vi "nanocal -- nuclear schottky fit V5.vi"() -> ()   [LabVIEW 2020] (continued)
"IDS0323_210901_RAW_cal__ref_"="IDS0323_210901_RAW_cal_CeCoIn5_4th_052(138)_C(f)_12T_3.10K_45deg_Tdep_raw_.dat", "IDS0323_210901_RAW_cal__sam_"="IDS0323_210901_RAW_cal_CeCoIn5_4th_052(138)_C(f)_12T_3.10K_45deg_Tdep_raw_.dat", "IDS0324_210901_RAW_cal__ref_"="IDS0324_210901_RAW_cal_CeCoIn5_4th_053(139)_C(f)_12T_5.70K_45deg_Tdep_raw_.dat", "IDS0324_210901_RAW_cal__sam_"="IDS0324_210901_RAW_cal_CeCoIn5_4th_053(139)_C(f)_12T_5.70K_45deg_Tdep_raw_.dat", "IDS0330_210901_RAW_cal__ref_"="IDS0330_210901_RAW_cal_CeCoIn5_4th_059_C(f)_1T_0.197K_90deg_Bdep_raw_.dat", "IDS0330_210901_RAW_cal__sam_"="IDS0330_210901_RAW_cal_CeCoIn5_4th_059_C(f)_1T_0.197K_90deg_Bdep_raw_.dat", "IDS0331_210901_RAW_cal__ref_"="IDS0331_210901_RAW_cal_CeCoIn5_4th_060_C(f)_2T_0.197K_90deg_Bdep_raw_.dat", "IDS0331_210901_RAW_cal__sam_"="IDS0331_210901_RAW_cal_CeCoIn5_4th_060_C(f)_2T_0.197K_90deg_Bdep_raw_.dat", "IDS0335_210904_RAW_cal__ref_"="IDS0335_210904_RAW_cal_CeCoIn5_4th_064_C(f)_5.0T_0.197K_90deg_fsweep_Tdep_raw_.dat", "IDS0335_210904_RAW_cal__sam_"="IDS0335_210904_RAW_cal_CeCoIn5_4th_064_C(f)_5.0T_0.197K_90deg_fsweep_Tdep_raw_.dat", "IDS0336_210904_RAW_cal__ref_"="IDS0336_210904_RAW_cal_CeCoIn5_4th_065_C(f)_5.0T_0.122K_90deg_fsweep_Tdep_raw_.dat", "IDS0336_210904_RAW_cal__sam_"="IDS0336_210904_RAW_cal_CeCoIn5_4th_065_C(f)_5.0T_0.122K_90deg_fsweep_Tdep_raw_.dat", "IDS0337_210904_RAW_cal__ref_"="IDS0337_210904_RAW_cal_CeCoIn5_4th_066_C(f)_5.0T_0.157K_90deg_Tdep_raw_.dat", "IDS0337_210904_RAW_cal__sam_"="IDS0337_210904_RAW_cal_CeCoIn5_4th_066_C(f)_5.0T_0.157K_90deg_Tdep_raw_.dat", "IDS0338_210904_RAW_cal__ref_"="IDS0338_210904_RAW_cal_CeCoIn5_4th_067_C(f)_5.0T_0.170K_90deg_Tdep_raw_.dat", "IDS0338_210904_RAW_cal__sam_"="IDS0338_210904_RAW_cal_CeCoIn5_4th_067_C(f)_5.0T_0.170K_90deg_Tdep_raw_.dat", "IDS0339_210904_RAW_cal__ref_"="IDS0339_210904_RAW_cal_CeCoIn5_4th_068_C(f)_5.0T_0.255K_90deg_Tdep_raw_.dat", "IDS0339_210904_RAW_cal__sam_"="IDS0339_210904_RAW_cal_CeCoIn5_4th_068_C(f)_5.0T_0.255K_90deg_Tdep_raw_.dat", "IDS0340_210904_RAW_cal__ref_"="IDS0340_210904_RAW_cal_CeCoIn5_4th_069_C(f)_5.0T_0.308K_90deg_Tdep_raw_.dat", "IDS0340_210904_RAW_cal__sam_"="IDS0340_210904_RAW_cal_CeCoIn5_4th_069_C(f)_5.0T_0.308K_90deg_Tdep_raw_.dat", "IDS0341_210904_RAW_cal__ref_"="IDS0341_210904_RAW_cal_CeCoIn5_4th_070_C(f)_5.0T_0.360K_90deg_Tdep_raw_.dat", "IDS0341_210904_RAW_cal__sam_"="IDS0341_210904_RAW_cal_CeCoIn5_4th_070_C(f)_5.0T_0.360K_90deg_Tdep_raw_.dat", "IDS0342_210904_RAW_cal__ref_"="IDS0342_210904_RAW_cal_CeCoIn5_4th_071_C(f)_5.0T_0.438K_90deg_Tdep_raw_.dat", "IDS0342_210904_RAW_cal__sam_"="IDS0342_210904_RAW_cal_CeCoIn5_4th_071_C(f)_5.0T_0.438K_90deg_Tdep_raw_.dat", "IDS0343_210904_RAW_cal__ref_"="IDS0343_210904_RAW_cal_CeCoIn5_4th_072_C(f)_5.0T_0.53K_90deg_Tdep_raw_.dat", "IDS0343_210904_RAW_cal__sam_"="IDS0343_210904_RAW_cal_CeCoIn5_4th_072_C(f)_5.0T_0.53K_90deg_Tdep_raw_.dat", "IDS0344_210904_RAW_cal__ref_"="IDS0344_210904_RAW_cal_CeCoIn5_4th_073_C(f)_5.0T_0.62K_90deg_Tdep_raw_.dat", "IDS0344_210904_RAW_cal__sam_"="IDS0344_210904_RAW_cal_CeCoIn5_4th_073_C(f)_5.0T_0.62K_90deg_Tdep_raw_.dat", "IDS0346_210904_RAW_cal__ref_"="IDS0346_210904_RAW_cal_CeCoIn5_4th_075_C(f)_8.0T_0.122K_90deg_Tdep_raw_.dat", "IDS0346_210904_RAW_cal__sam_"="IDS0346_210904_RAW_cal_CeCoIn5_4th_075_C(f)_8.0T_0.122K_90deg_Tdep_raw_.dat", "IDS0347_210906_RAW_cal__ref_"="IDS0347_210906_RAW_cal_CeCoIn5_4th_076_C(f)_8.0T_0.157K_90deg_Tdep_raw_.dat", "IDS0347_210906_RAW_cal__sam_"="IDS0347_210906_RAW_cal_CeCoIn5_4th_076_C(f)_8.0T_0.157K_90deg_Tdep_raw_.dat", "IDS0348_210906_RAW_cal__ref_"="IDS0348_210906_RAW_cal_CeCoIn5_4th_077_C(f)_8.0T_0.178K_90deg_Tdep_raw_.dat", "IDS0348_210906_RAW_cal__sam_"="IDS0348_210906_RAW_cal_CeCoIn5_4th_077_C(f)_8.0T_0.178K_90deg_Tdep_raw_.dat", "IDS0349_210906_RAW_cal__ref_"="IDS0349_210906_RAW_cal_CeCoIn5_4th_078_C(f)_8.0T_0.20K_90deg_Tdep_raw_.dat", "IDS0349_210906_RAW_cal__sam_"="IDS0349_210906_RAW_cal_CeCoIn5_4th_078_C(f)_8.0T_0.20K_90deg_Tdep_raw_.dat", "IDS0350_210906_RAW_cal__ref_"="IDS0350_210906_RAW_cal_CeCoIn5_4th_079_C(f)_8.0T_0.26K_90deg_Tdep_raw_.dat", "IDS0350_210906_RAW_cal__sam_"="IDS0350_210906_RAW_cal_CeCoIn5_4th_079_C(f)_8.0T_0.26K_90deg_Tdep_raw_.dat", "IDS0351_210906_RAW_cal__ref_"="IDS0351_210906_RAW_cal_CeCoIn5_4th_080_C(f)_8.0T_0.31K_90deg_Tdep_raw_.dat", "IDS0351_210906_RAW_cal__sam_"="IDS0351_210906_RAW_cal_CeCoIn5_4th_080_C(f)_8.0T_0.31K_90deg_Tdep_raw_.dat", "IDS0352_210906_RAW_cal__ref_"="IDS0352_210906_RAW_cal_CeCoIn5_4th_081_C(f)_8.0T_0.36K_90deg_Tdep_raw_.dat", "IDS0352_210906_RAW_cal__sam_"="IDS0352_210906_RAW_cal_CeCoIn5_4th_081_C(f)_8.0T_0.36K_90deg_Tdep_raw_.dat", "IDS0353_210906_RAW_cal__ref_"="IDS0353_210906_RAW_cal_CeCoIn5_4th_082_C(f)_8.0T_0.438K_90deg_Tdep_raw_.dat", "IDS0353_210906_RAW_cal__sam_"="IDS0353_210906_RAW_cal_CeCoIn5_4th_082_C(f)_8.0T_0.438K_90deg_Tdep_raw_.dat", "IDS0354_210906_RAW_cal__ref_"="IDS0354_210906_RAW_cal_CeCoIn5_4th_083_C(f)_8.0T_0.53K_90deg_Tdep_raw_.dat", "IDS0354_210906_RAW_cal__sam_"="IDS0354_210906_RAW_cal_CeCoIn5_4th_083_C(f)_8.0T_0.53K_90deg_Tdep_raw_.dat", "IDS0355_210906_RAW_cal__ref_"="IDS0355_210906_RAW_cal_CeCoIn5_4th_085_C(f)_8.0T_0.83K_90deg_Tdep_raw_.dat", "IDS0355_210906_RAW_cal__sam_"="IDS0355_210906_RAW_cal_CeCoIn5_4th_085_C(f)_8.0T_0.83K_90deg_Tdep_raw_.dat", "IDS0359_210907_RAW_cal__ref_"="IDS0359_210907_RAW_cal_CeCoIn5_4th_089_C(f)_12.0T_0.12K_60deg_Tdep_raw_.dat", "IDS0359_210907_RAW_cal__sam_"="IDS0359_210907_RAW_cal_CeCoIn5_4th_089_C(f)_12.0T_0.12K_60deg_Tdep_raw_.dat", "IDS0360_210907_RAW_cal__ref_"="IDS0360_210907_RAW_cal_CeCoIn5_4th_090_C(f)_12.0T_0.15K_60deg_Tdep_raw_.dat", "IDS0360_210907_RAW_cal__sam_"="IDS0360_210907_RAW_cal_CeCoIn5_4th_090_C(f)_12.0T_0.15K_60deg_Tdep_raw_.dat", "IDS0361_210908_RAW_cal__ref_"="IDS0361_210908_RAW_cal_CeCoIn5_4th_091_C(f)_12.0T_0.168K_60deg_Tdep_raw_.dat", "IDS0361_210908_RAW_cal__sam_"="IDS0361_210908_RAW_cal_CeCoIn5_4th_091_C(f)_12.0T_0.168K_60deg_Tdep_raw_.dat", "IDS0362_210908_RAW_cal__ref_"="IDS0362_210908_RAW_cal_CeCoIn5_4th_092_C(f)_12.0T_0.197K_60deg_Tdep_raw_.dat", "IDS0362_210908_RAW_cal__sam_"="IDS0362_210908_RAW_cal_CeCoIn5_4th_092_C(f)_12.0T_0.197K_60deg_Tdep_raw_.dat", "IDS0363_210908_RAW_cal__ref_"="IDS0363_210908_RAW_cal_CeCoIn5_4th_093_C(f)_12.0T_0.25K_60deg_Tdep_raw_.dat", "IDS0363_210908_RAW_cal__sam_"="IDS0363_210908_RAW_cal_CeCoIn5_4th_093_C(f)_12.0T_0.25K_60deg_Tdep_raw_.dat", "IDS0364_210908_RAW_cal__ref_"="IDS0364_210908_RAW_cal_CeCoIn5_4th_094_C(f)_12.0T_0.307K_60deg_Tdep_raw_.dat", "IDS0364_210908_RAW_cal__sam_"="IDS0364_210908_RAW_cal_CeCoIn5_4th_094_C(f)_12.0T_0.307K_60deg_Tdep_raw_.dat", "IDS0365_210908_RAW_cal__ref_"="IDS0365_210908_RAW_cal_CeCoIn5_4th_095_C(f)_12.0T_0.36K_60deg_Tdep_raw_.dat", "IDS0365_210908_RAW_cal__sam_"="IDS0365_210908_RAW_cal_CeCoIn5_4th_095_C(f)_12.0T_0.36K_60deg_Tdep_raw_.dat", "IDS0366_210908_RAW_cal__ref_"="IDS0366_210908_RAW_cal_CeCoIn5_4th_096_C(f)_12.0T_0.43K_60deg_Tdep_raw_.dat", "IDS0366_210908_RAW_cal__sam_"="IDS0366_210908_RAW_cal_CeCoIn5_4th_096_C(f)_12.0T_0.43K_60deg_Tdep_raw_.dat", "IDS0367_210908_RAW_cal__ref_"="IDS0367_210908_RAW_cal_CeCoIn5_4th_097_C(f)_12.0T_0.53K_60deg_Tdep_raw_.dat", "IDS0367_210908_RAW_cal__sam_"="IDS0367_210908_RAW_cal_CeCoIn5_4th_097_C(f)_12.0T_0.53K_60deg_Tdep_raw_.dat", "IDS0368_210908_RAW_cal__ref_"="IDS0368_210908_RAW_cal_CeCoIn5_4th_098_C(f)_12.0T_0.63K_60deg_Tdep_raw_.dat", "IDS0368_210908_RAW_cal__sam_"="IDS0368_210908_RAW_cal_CeCoIn5_4th_098_C(f)_12.0T_0.63K_60deg_Tdep_raw_.dat", "IDS0369_210908_RAW_cal__ref_"="IDS0369_210908_RAW_cal_CeCoIn5_4th_099_C(f)_12.0T_0.83K_60deg_Tdep_raw_.dat", "IDS0369_210908_RAW_cal__sam_"="IDS0369_210908_RAW_cal_CeCoIn5_4th_099_C(f)_12.0T_0.83K_60deg_Tdep_raw_.dat", "IDS0370_210908_RAW_cal__ref_"="IDS0370_210908_RAW_cal_CeCoIn5_4th_100_C(f)_12.0T_1.13K_60deg_Tdep_raw_.dat", "IDS0370_210908_RAW_cal__sam_"="IDS0370_210908_RAW_cal_CeCoIn5_4th_100_C(f)_12.0T_1.13K_60deg_Tdep_raw_.dat", "IDS0371_210908_RAW_cal__ref_"="IDS0371_210908_RAW_cal_CeCoIn5_4th_101_C(f)_12.0T_1.90K_60deg_Tdep_raw_.dat", "IDS0371_210908_RAW_cal__sam_"="IDS0371_210908_RAW_cal_CeCoIn5_4th_101_C(f)_12.0T_1.90K_60deg_Tdep_raw_.dat", "IDS0372_210908_RAW_cal__ref_"="IDS0372_210908_RAW_cal_CeCoIn5_4th_102_C(f)_12.0T_3.11K_60deg_Tdep_raw_.dat", "IDS0372_210908_RAW_cal__sam_"="IDS0372_210908_RAW_cal_CeCoIn5_4th_102_C(f)_12.0T_3.11K_60deg_Tdep_raw_.dat", "IDS0373_210908_RAW_cal__ref_"="IDS0373_210908_RAW_cal_CeCoIn5_4th_103_C(f)_12.0T_5.75K_60deg_Tdep_raw_.dat", "IDS0373_210908_RAW_cal__sam_"="IDS0373_210908_RAW_cal_CeCoIn5_4th_103_C(f)_12.0T_5.75K_60deg_Tdep_raw_.dat", "IDS0377_210909_RAW_cal__ref_"="IDS0377_210909_RAW_cal_CeCoIn5_4th_107_C(f)_8.0T_0.197K_0deg_Tdep_raw_.dat", "IDS0377_210909_RAW_cal__sam_"="IDS0377_210909_RAW_cal_CeCoIn5_4th_107_C(f)_8.0T_0.197K_0deg_Tdep_raw_.dat", "IDS0378_210909_RAW_cal__ref_"="IDS0378_210909_RAW_cal_CeCoIn5_4th_108_C(f)_8.0T_0.122K_0deg_Tdep_raw_.dat", "IDS0378_210909_RAW_cal__sam_"="IDS0378_210909_RAW_cal_CeCoIn5_4th_108_C(f)_8.0T_0.122K_0deg_Tdep_raw_.dat", "IDS0379_210909_RAW_cal__ref_"="IDS0379_210909_RAW_cal_CeCoIn5_4th_109_C(f)_8.0T_0.148K_0deg_Tdep_raw_.dat", "IDS0379_210909_RAW_cal__sam_"="IDS0379_210909_RAW_cal_CeCoIn5_4th_109_C(f)_8.0T_0.148K_0deg_Tdep_raw_.dat", "IDS0380_210909_RAW_cal__ref_"="IDS0380_210909_RAW_cal_CeCoIn5_4th_110_C(f)_8.0T_0.168K_0deg_Tdep_raw_.dat", "IDS0380_210909_RAW_cal__sam_"="IDS0380_210909_RAW_cal_CeCoIn5_4th_110_C(f)_8.0T_0.168K_0deg_Tdep_raw_.dat", "IDS0381_210909_RAW_cal__ref_"="IDS0381_210909_RAW_cal_CeCoIn5_4th_111_C(f)_8.0T_0.25K_0deg_Tdep_raw_.dat", "IDS0381_210909_RAW_cal__sam_"="IDS0381_210909_RAW_cal_CeCoIn5_4th_111_C(f)_8.0T_0.25K_0deg_Tdep_raw_.dat", "IDS0382_210909_RAW_cal__ref_"="IDS0382_210909_RAW_cal_CeCoIn5_4th_112_C(f)_8.0T_0.30K_0deg_Tdep_raw_.dat", "IDS0382_210909_RAW_cal__sam_"="IDS0382_210909_RAW_cal_CeCoIn5_4th_112_C(f)_8.0T_0.30K_0deg_Tdep_raw_.dat", "IDS0383_210910_RAW_cal__ref_"="IDS0383_210910_RAW_cal_CeCoIn5_4th_113_C(f)_8.0T_0.36K_0deg_Tdep_raw_.dat", "IDS0383_210910_RAW_cal__sam_"="IDS0383_210910_RAW_cal_CeCoIn5_4th_113_C(f)_8.0T_0.36K_0deg_Tdep_raw_.dat", "IDS0384_210910_RAW_cal__ref_"="IDS0384_210910_RAW_cal_CeCoIn5_4th_114_C(f)_8.0T_0.43K_0deg_Tdep_raw_.dat", "IDS0384_210910_RAW_cal__sam_"="IDS0384_210910_RAW_cal_CeCoIn5_4th_114_C(f)_8.0T_0.43K_0deg_Tdep_raw_.dat", "IDS0385_210910_RAW_cal__ref_"="IDS0385_210910_RAW_cal_CeCoIn5_4th_115_C(f)_8.0T_0.53K_0deg_Tdep_raw_.dat", "IDS0385_210910_RAW_cal__sam_"="IDS0385_210910_RAW_cal_CeCoIn5_4th_115_C(f)_8.0T_0.53K_0deg_Tdep_raw_.dat", "IDS0386_210910_RAW_cal__ref_"="IDS0386_210910_RAW_cal_CeCoIn5_4th_116_C(f)_8.0T_0.63K_0deg_Tdep_raw_.dat", "IDS0386_210910_RAW_cal__sam_"="IDS0386_210910_RAW_cal_CeCoIn5_4th_116_C(f)_8.0T_0.63K_0deg_Tdep_raw_.dat", "IDS0387_210910_RAW_cal__ref_"="IDS0387_210910_RAW_cal_CeCoIn5_4th_117_C(f)_8.0T_0.83K_0deg_Tdep_raw_.dat", "IDS0387_210910_RAW_cal__sam_"="IDS0387_210910_RAW_cal_CeCoIn5_4th_117_C(f)_8.0T_0.83K_0deg_Tdep_raw_.dat", "IDS0388_210910_RAW_cal__ref_"="IDS0388_210910_RAW_cal_CeCoIn5_4th_118_C(f)_8.0T_1.13K_0deg_Tdep_raw_.dat", "IDS0388_210910_RAW_cal__sam_"="IDS0388_210910_RAW_cal_CeCoIn5_4th_118_C(f)_8.0T_1.13K_0deg_Tdep_raw_.dat", "IDS0389_210910_RAW_cal__ref_"="IDS0389_210910_RAW_cal_CeCoIn5_4th_119_C(f)_8.0T_1.52K_0deg_Tdep_raw_.dat", "IDS0389_210910_RAW_cal__sam_"="IDS0389_210910_RAW_cal_CeCoIn5_4th_119_C(f)_8.0T_1.52K_0deg_Tdep_raw_.dat", "IDS0390_210910_RAW_cal__ref_"="IDS0390_210910_RAW_cal_CeCoIn5_4th_120_C(f)_8.0T_1.90K_0deg_Tdep_raw_.dat", "IDS0390_210910_RAW_cal__sam_"="IDS0390_210910_RAW_cal_CeCoIn5_4th_120_C(f)_8.0T_1.90K_0deg_Tdep_raw_.dat", "IDS0391_210910_RAW_cal__ref_"="IDS0391_210910_RAW_cal_CeCoIn5_4th_121_C(f)_8.0T_1.25K_0deg_Tdep_raw_.dat", "IDS0391_210910_RAW_cal__sam_"="IDS0391_210910_RAW_cal_CeCoIn5_4th_121_C(f)_8.0T_1.25K_0deg_Tdep_raw_.dat", "IDS0392_210910_RAW_cal__ref_"="IDS0392_210910_RAW_cal_CeCoIn5_4th_122_C(f)_8.0T_1.39K_0deg_Tdep_raw_.dat", "IDS0392_210910_RAW_cal__sam_"="IDS0392_210910_RAW_cal_CeCoIn5_4th_122_C(f)_8.0T_1.39K_0deg_Tdep_raw_.dat", "IDS0393_210910_RAW_cal__ref_"="IDS0393_210910_RAW_cal_CeCoIn5_4th_123_C(f)_8.0T_3.11K_0deg_Tdep_raw_.dat", "IDS0393_210910_RAW_cal__sam_"="IDS0393_210910_RAW_cal_CeCoIn5_4th_123_C(f)_8.0T_3.11K_0deg_Tdep_raw_.dat", "IDS0394_210910_RAW_cal__ref_"="IDS0394_210910_RAW_cal_CeCoIn5_4th_124_C(f)_8.0T_5.75K_0deg_Tdep_raw_.dat", "IDS0394_210910_RAW_cal__sam_"="IDS0394_210910_RAW_cal_CeCoIn5_4th_124_C(f)_8.0T_5.75K_0deg_Tdep_raw_.dat", "IDS0395_210910_RAW_cal__ref_"="IDS0395_210910_RAW_cal_CeCoIn5_4th_125_C(f)_8.0T_1.31K_0deg_Tdep_raw_.dat", "IDS0395_210910_RAW_cal__sam_"="IDS0395_210910_RAW_cal_CeCoIn5_4th_125_C(f)_8.0T_1.31K_0deg_Tdep_raw_.dat"}
  out "temps&degs":map{string, map{T4, dbl}}(c390)
  out "mathematica thing":map{string, map{T4, dbl}}(c390)
  out "constrained filename lookup":map{i32, string}(c390)={0="IDS0336_210904_RAW_cal__ref_", 1="IDS0337_210904_RAW_cal__ref_", 2="IDS0338_210904_RAW_cal__ref_", 3="IDS0335_210904_RAW_cal__ref_", 4="IDS0339_210904_RAW_cal__ref_", 5="IDS0340_210904_RAW_cal__ref_", 6="IDS0341_210904_RAW_cal__ref_", 7="IDS0342_210904_RAW_cal__ref_", 8="IDS0343_210904_RAW_cal__ref_", 9="IDS0344_210904_RAW_cal__ref_"}
  out "filesnames lookup":map{i32, string}(c390)={0="IDS0183_210310_RAW_cal__sam_", 1="IDS0311_210901_RAW_cal__sam_", 2="IDS0359_210907_RAW_cal__sam_", 3="IDS0336_210904_RAW_cal__sam_", 4="IDS0346_210904_RAW_cal__sam_", 5="IDS0378_210909_RAW_cal__sam_", 6="IDS0158_210310_RAW_cal__sam_", 7="IDS0300_210427_RAW_cal__sam_", 8="IDS0184_210310_RAW_cal__sam_", 9="IDS0210_210310_RAW_cal__sam_", 10="IDS0379_210909_RAW_cal__sam_", 11="IDS0360_210907_RAW_cal__sam_", 12="IDS0310_210901_RAW_cal__sam_", 13="IDS0337_210904_RAW_cal__sam_", 14="IDS0347_210906_RAW_cal__sam_", 15="IDS0305_210831_RAW_cal__sam_", 16="IDS0361_210908_RAW_cal__sam_", 17="IDS0380_210909_RAW_cal__sam_", 18="IDS0159_210310_RAW_cal__sam_", 19="IDS0304_210831_RAW_cal__sam_", 20="IDS0312_210901_RAW_cal__sam_", 21="IDS0338_210904_RAW_cal__sam_", 22="IDS0348_210906_RAW_cal__sam_", 23="IDS0181_210310_RAW_cal__sam_", 24="IDS0185_210310_RAW_cal__sam_", 25="IDS0208_210310_RAW_cal__sam_", 26="IDS0209_210310_RAW_cal__sam_", 27="IDS0211_210310_RAW_cal__sam_", 28="IDS0212_210310_RAW_cal__sam_", 29="IDS0213_210310_RAW_cal__sam_", 30="IDS0214_210310_RAW_cal__sam_", 31="IDS0215_210310_RAW_cal__sam_", 32="IDS0216_210310_RAW_cal__sam_", 33="IDS0217_210310_RAW_cal__sam_", 34="IDS0330_210901_RAW_cal__sam_", 35="IDS0331_210901_RAW_cal__sam_", 36="IDS0335_210904_RAW_cal__sam_", 37="IDS0362_210908_RAW_cal__sam_", 38="IDS0377_210909_RAW_cal__sam_", 39="IDS0160_210310_RAW_cal__sam_", 40="IDS0303_210831_RAW_cal__sam_", 41="IDS0313_210901_RAW_cal__sam_", 42="IDS0349_210906_RAW_cal__sam_", 43="IDS0161_210310_RAW_cal__sam_", 44="IDS0186_210310_RAW_cal__sam_", 45="IDS0302_210831_RAW_cal__sam_", 46="IDS0363_210908_RAW_cal__sam_", 47="IDS0381_210909_RAW_cal__sam_", 48="IDS0314_210901_RAW_cal__sam_", 49="IDS0339_210904_RAW_cal__sam_", 50="IDS0350_210906_RAW_cal__sam_", 51="IDS0162_210310_RAW_cal__sam_", 52="IDS0187_210310_RAW_cal__sam_", 53="IDS0301_210831_RAW_cal__sam_", 54="IDS0315_210901_RAW_cal__sam_", 55="IDS0382_210909_RAW_cal__sam_", 56="IDS0364_210908_RAW_cal__sam_", 57="IDS0340_210904_RAW_cal__sam_", 58="IDS0351_210906_RAW_cal__sam_", 59="IDS0163_210310_RAW_cal__sam_", 60="IDS0188_210310_RAW_cal__sam_", 61="IDS0299_210427_RAW_cal__sam_", 62="IDS0316_210901_RAW_cal__sam_", 63="IDS0341_210904_RAW_cal__sam_", 64="IDS0352_210906_RAW_cal__sam_", 65="IDS0365_210908_RAW_cal__sam_", 66="IDS0383_210910_RAW_cal__sam_", 67="IDS0164_210310_RAW_cal__sam_", 68="IDS0189_210310_RAW_cal__sam_", 69="IDS0298_210427_RAW_cal__sam_", 70="IDS0317_210901_RAW_cal__sam_", 71="IDS0366_210908_RAW_cal__sam_", 72="IDS0384_210910_RAW_cal__sam_", 73="IDS0342_210904_RAW_cal__sam_", 74="IDS0353_210906_RAW_cal__sam_", 75="IDS0165_210310_RAW_cal__sam_", 76="IDS0190_210310_RAW_cal__sam_", 77="IDS0297_210427_RAW_cal__sam_", 78="IDS0318_210901_RAW_cal__sam_", 79="IDS0343_210904_RAW_cal__sam_", 80="IDS0354_210906_RAW_cal__sam_", 81="IDS0367_210908_RAW_cal__sam_", 82="IDS0385_210910_RAW_cal__sam_", 83="IDS0166_210310_RAW_cal__sam_", 84="IDS0191_210310_RAW_cal__sam_", 85="IDS0296_210427_RAW_cal__sam_", 86="IDS0319_210901_RAW_cal__sam_", 87="IDS0344_210904_RAW_cal__sam_", 88="IDS0368_210908_RAW_cal__sam_", 89="IDS0386_210910_RAW_cal__sam_", 90="IDS0220_210310_RAW_cal__sam_", 91="IDS0167_210310_RAW_cal__sam_", 92="IDS0192_210310_RAW_cal__sam_", 93="IDS0295_210427_RAW_cal__sam_", 94="IDS0320_210901_RAW_cal__sam_", 95="IDS0355_210906_RAW_cal__sam_", 96="IDS0369_210908_RAW_cal__sam_", 97="IDS0387_210910_RAW_cal__sam_", 98="IDS0168_210310_RAW_cal__sam_", 99="IDS0219_210310_RAW_cal__sam_", 100="IDS0193_210310_RAW_cal__sam_", 101="IDS0294_210427_RAW_cal__sam_", 102="IDS0321_210901_RAW_cal__sam_", 103="IDS0370_210908_RAW_cal__sam_", 104="IDS0388_210910_RAW_cal__sam_", 105="IDS0169_210310_RAW_cal__sam_", 106="IDS0391_210910_RAW_cal__sam_", 107="IDS0395_210910_RAW_cal__sam_", 108="IDS0392_210910_RAW_cal__sam_", 109="IDS0389_210910_RAW_cal__sam_", 110="IDS0218_210310_RAW_cal__sam_", 111="IDS0194_210310_RAW_cal__sam_", 112="IDS0293_210427_RAW_cal__sam_", 113="IDS0322_210901_RAW_cal__sam_", 114="IDS0371_210908_RAW_cal__sam_", 115="IDS0390_210910_RAW_cal__sam_", 116="IDS0170_210310_RAW_cal__sam_", 117="IDS0195_210310_RAW_cal__sam_", 118="IDS0306_210831_RAW_cal__sam_", 119="IDS0323_210901_RAW_cal__sam_", 120="IDS0372_210908_RAW_cal__sam_", 121="IDS0393_210910_RAW_cal__sam_", 122="IDS0171_210310_RAW_cal__sam_", 123="IDS0196_210310_RAW_cal__sam_", 124="IDS0324_210901_RAW_cal__sam_", 125="IDS0373_210908_RAW_cal__sam_", 126="IDS0394_210910_RAW_cal__sam_", 127="IDS0172_210310_RAW_cal__sam_"}
  in  "parameter map":map{T4, dbl}(c390)={enum."ζ"=0.2919164673041952, enum."τ1"=0.04813472468486327, enum."τS"=0.13257313400894957, enum."τN"=0.017459219246992615, enum."τC"=0.0011273379303887484, enum."κ0"=6.401291929673956e-10}
  out "all full filenames":map{string, path}(c390)
  in  "tab 9":enum32{"Page 1"}(tab)
  in  "# plot steps":i32=200
  out "Plot: oscillations":cluster{"Array":i32[], "Array":dbl[]}(graph)={"Array"=[0, 1, 2, 3, 4, 5, 6, 7, 8, 9, 10, 11, 12, 13, 14, 15, 16, 17, 18, 19, 20, 21, 22, 23, 24, 25, 26, 27, 28, 29, 30, 31, 32, 33, 34, 35, 36, 37, 38, 39, 40, 41, 42, 43, 44, 45, 46, 47, 48, 49, 50, 51, 52, 53, 54, 55, 56, 57, 58, 59, 60, 61, 62, 63, 64, 65, 66, 67, 68, 69, 70, 71, 72, 73, 74, 75, 76, 77, 78, 79, 80, 81, 82, 83, 84, 85, 86, 87, 88, 89, 90, 91, 92, 93, 94, 95, 96, 97, 98, 99, 100, 101, 102, 103, 104, 105, 106, 107, 108, 109, 110, 111, 112, 113, 114, 115, 116, 117, 118, 119, 120, 121, 122, 123, 124, 125, 126, 127, 128, 129, 130, 131, 132, 133, 134, 135, 136, 137, 138, 139, 140, 141, 142, 143, 144, 145, 146, 147, 148, 149, 150, 151, 152, 153, 154, 155, 156, 157, 158, 159, 160, 161, 162, 163, 164, 165, 166, 167, 168, 169, 170, 171, 172, 173, 174, 175, 176, 177, 178, 179, 180, 181, 182, 183, 184, 185, 186, 187, 188, 189, 190, 191, 192, 193, 194, 195, 196, 197, 198, 199], "Array"=[4.450467078198628e-11, 4.3160530704966504e-11, 4.183009494340695e-11, 4.0513266352792954e-11, 3.9210031055336714e-11, 3.792043068440165e-11, 3.664459014007804e-11, 3.5382301255548754e-11, 3.413366811422236e-11, 3.2898669899417143e-11, 3.167733436670872e-11, 3.0469723966142226e-11, 2.927564440868835e-11, 2.8095047122089767e-11, 2.6928285989935574e-11, 2.5775048762000097e-11, 2.4635564421782163e-11, 2.3509562352419522e-11, 2.239730623188052e-11, 2.1298608710029754e-11, 2.0213615503639204e-11, 1.9142160079255177e-11, 1.8084339581392328e-11, 1.704010543779333e-11, 1.600961724301797e-11, 1.4992611319097904e-11, 1.3989330527319765e-11, 1.2999573639760342e-11, 1.2023514128767232e-11, 1.106102015535626e-11, 1.0112154169572563e-11, 9.176874538052715e-12, 8.25520207747843e-12, 7.347261687939977e-12, 6.452831324832431e-12, 5.572056704927775e-12, 4.704805989241834e-12, 3.8511763222892625e-12, 3.0112856652664277e-12, 2.1848217679476534e-12, 1.3720968805586153e-12, 5.7278487508583e-13, -2.1275342598769953e-13, -9.847817006303217e-13, -1.743175048751766e-12, -2.4878918369886094e-12, -3.2191541099457766e-12, -3.936725945230535e-12, -4.6408710208112325e-12, -5.331263208674386e-12, -6.0080551644858815e-12, -6.671233010457911e-12, -7.32107430234663e-12, -7.957107195366575e-12, -8.579630061955612e-12, -9.188531879811279e-12, -9.783868160084808e-12, -1.0365638902776197e-11, -1.0933837168991545e-11, -1.1488317241958867e-11, -1.2029287288495283e-11, -1.2556754247494695e-11, -1.3070614035548545e-11, -1.3570831958187313e-11, -1.4057588426652501e-11, -1.453061976297576e-11, -1.4990300667427903e-11, -1.5436249500844212e-11, -1.586871606340523e-11, -1.628758239391459e-11, -1.6692904003523523e-11, -1.7084472725414912e-11, -1.7462697954329087e-11, -1.7827309073403796e-11, -1.8178437921623214e-11, -1.851580000433728e-11, -1.883979777739242e-11, -1.9150098173881247e-11, -1.9447013444029437e-11, -1.9730182765353987e-11, -1.9999855938035438e-11, -2.0255956634240846e-11, -2.0498630570742193e-11, -2.0727621008465036e-11, -2.094310141975697e-11, -2.1145078743511903e-11, -2.133339338517004e-11, -2.15082465726546e-11, -2.1669575855920442e-11, -2.1817395112755378e-11, -2.1951523931917905e-11, -2.20721010912861e-11, -2.2179251490950236e-11, -2.2272947375334695e-11, -2.2352932005365034e-11, -2.241937885338885e-11, -2.2472315674981758e-11, -2.251185349244622e-11, -2.25377425056017e-11, -2.2550079858962846e-11, -2.2548990452619933e-11, -2.2534259180861937e-11, -2.2506121966081594e-11, -2.2464322069204457e-11, -2.2409005207002508e-11, -2.234022689062698e-11, -2.2257855281093697e-11, -2.2161987522917315e-11, -2.205260279941612e-11, -2.192974274395354e-11, -2.179331715090882e-11, -2.164343010369052e-11, -2.1479908129951042e-11, -2.1302994090977023e-11, -2.111255614778429e-11, -2.090846940028257e-11, -2.0690962831970694e-11, -2.0459987870591334e-11, -2.0215468188311547e-11, -1.9957403785131334e-11, -1.9685864049989732e-11, -1.9400814288417223e-11, -1.9102282255989422e-11, -1.8790205502661195e-11, -1.8464556272856925e-11, -1.812547334445469e-11, -1.777293590077278e-11, -1.7406853736190442e-11, -1.7027261545177197e-11, -1.66342564722477e-11, -1.6227671983948255e-11, -1.5807473385809345e-11, -1.5374167217085954e-11, -1.492703877170598e-11, -1.4466448872152426e-11, -1.399237670174358e-11, -1.3504822260479443e-11, -1.3003882692874669e-11, -1.248931513764262e-11, -1.1961341639388223e-11, -1.1419837298021207e-11, -1.0864954769207458e-11, -1.029650670281157e-11, -9.714548609984774e-12, -9.119142940772207e-12, -8.510296634067771e-12, -7.88796111761414e-12, -7.252087819153985e-12, -6.60278776098977e-12, -5.939956859712936e-12, -5.263699198732041e-12, -4.573903755744624e-12, -3.870841147612936e-12, -3.1540256517637033e-12, -2.423963807451912e-12, -1.6803017310884627e-12, -9.233377951112232e-13, -1.5276668818842154e-13, 6.312797506957679e-13, 1.428669682557171e-12, 2.2397153576214635e-12, 3.0641184034507774e-12, 3.901934331196344e-12, 4.7532186520093944e-12, 5.618054632616776e-12, 6.496254922883082e-12, 7.387951361792489e-12, 8.293039865936436e-12, 9.211555129784443e-12, 1.014360123674507e-11, 1.108921982018174e-11, 1.2048202713277334e-11, 1.3020501343774527e-11, 1.400635163406605e-11, 1.5005753584151904e-11, 1.601835331044299e-11, 1.7044518574316214e-11, 1.808416610904473e-11, 1.9137177953432172e-11, 2.0203720640932232e-11, 2.1283551310258275e-11, 2.237704466168111e-11, 2.3483812117142122e-11, 2.4604082660140136e-11, 2.573779384063002e-11, 2.688487626967273e-11, 2.8045406275101215e-11, 2.921947406253622e-11, 3.0406781259539883e-11, 3.160766093301959e-11, 3.282196042730945e-11, 3.4049658925727755e-11, 3.5290666222653755e-11, 3.654530844610093e-11, 3.781320395690457e-11, 3.909453316630618e-11, 4.03893932188204e-11, 4.169764533656917e-11, 4.3019296458446377e-11, 4.435427719551299e-11]}
  out "current step ind":i32=16574
  out "current plot ind":i32=166
  out "|v_i| = | dlogG/dlogα_i | (log scale slider)":dbl[](array[slide])=[3.065919719494306e-06, 0.0007578980980653129, 7.802452151739537e-05, 0.0005349845415649405, 7.224415710242577e-07, 2.2288197381997078e-07] scale=1e-08..10.0 scale format="%#_2p"
  in  "total # steps":i32=50000
  in  "update rate":i32=100
  out "side map from NUM":map{i32, T11}(c390)={4000=enum."ref", 8000=enum."sam"}
  out "side map to STR":map{T11, string}(c390)={enum."sam"="_sam_", enum."ref"="_ref_"}
  out "side map to NUM":map{T11, i32}(c390)={enum."sam"=8000, enum."ref"=4000}
  out "data file parameters map":map{T4, T12}(c390)={enum."T (K)"=enum."get T", enum."B (T)"=enum."get B", enum."θ (deg)"=enum."get deg", enum."set of (B|T)"=enum."get change"}
  in  "cursor index map":map{T4, i32}(c390)={enum."ζ"=0, enum."τ1"=1, enum."τS"=2, enum."τN"=3, enum."τC"=4, enum."κ0"=5, enum."m1"=6, enum."m2"=7, enum."m3"=8}
  out "new selector names":map{T4, map{T13, string}}(c390)={enum."ζ"={enum."name"="ζ", enum."nameL"="zeta", enum."units"="sec", enum."prec"="%_4p"}, enum."τ1"={enum."name"="τ1", enum."nameL"="tau1", enum."units"="sec", enum."prec"="%_4p"}, enum."τS"={enum."name"="τS", enum."nameL"="tauS", enum."units"="sec", enum."prec"="%_4p"}, enum."τN"={enum."name"="τN", enum."nameL"="tauN", enum."units"="sec", enum."prec"="%_4p"}, enum."τC"={enum."name"="τC", enum."nameL"="tauC", enum."units"="sec", enum."prec"="%_4p"}, enum."κ0"={enum."name"="κ0", enum."nameL"="kappa0", enum."units"="WperK", enum."prec"="%_5p"}, enum."T (K)"={enum."name"="T", enum."nameL"="T", enum."units"="K", enum."prec"="%_4p"}, enum."B (T)"={enum."name"="B", enum."nameL"="B", enum."units"="T", enum."prec"="%_2p"}, enum."θ (deg)"={enum."name"="θ", enum."nameL"="theta", enum."units"="deg", enum."prec"="%_2p"}, enum."side (S|R)"={enum."name"="side", enum."nameL"="side", enum."units"="side", enum."prec"="%d"}}
  out "state of all selectors string":string="__5.0T__90deg__4000side_"
  out "state of all selectors":map{T4, map{bool, dbl}}(c390)={enum."T (K)"={TRUE=0.179}, enum."B (T)"={FALSE=5.0}, enum."θ (deg)"={FALSE=90.0}, enum."side (S|R)"={FALSE=4000.0}, enum."set of (B|T)"={FALSE=1.0}}
  in  "reverse cursor index map":map{i32, T4}(c390)={0=enum."ζ", 1=enum."τ1", 2=enum."τS", 3=enum."τN", 4=enum."τC", 5=enum."κ0", 6=enum."m1", 7=enum."m2", 8=enum."m3"}
  in  "tab 7":enum32{"Page 1"}(tab)
  in  "tab 3":enum32{"Page 1"}(tab)
  out "key":string="IDS0337_210904_RAW_cal__ref_"
  out "T (K)":dbl=0.157 format="%#_10f"
  out "θ (deg)":dbl=90.0 format="%#_10f"
  out "B (T)":dbl=5.0
  in  "tab 6":enum32{"Page 1"}(tab)
  in  "τ→Math! :p":bool
  in  "selection :|\\":u16(ring)=1 caption="files" items=["IDS0336_210904_RAW_cal_CeCoIn5_4th_065_C(f)_5.0T_0.122K_90deg_fsweep_Tdep_raw_.dat", "IDS0337_210904_RAW_cal_CeCoIn5_4th_066_C(f)_5.0T_0.157K_90deg_Tdep_raw_.dat", "IDS0338_210904_RAW_cal_CeCoIn5_4th_067_C(f)_5.0T_0.170K_90deg_Tdep_raw_.dat", "IDS0335_210904_RAW_cal_CeCoIn5_4th_064_C(f)_5.0T_0.197K_90deg_fsweep_Tdep_raw_.dat", "IDS0339_210904_RAW_cal_CeCoIn5_4th_068_C(f)_5.0T_0.255K_90deg_Tdep_raw_.dat", "IDS0340_210904_RAW_cal_CeCoIn5_4th_069_C(f)_5.0T_0.308K_90deg_Tdep_raw_.dat", "IDS0341_210904_RAW_cal_CeCoIn5_4th_070_C(f)_5.0T_0.360K_90deg_Tdep_raw_.dat", "IDS0342_210904_RAW_cal_CeCoIn5_4th_071_C(f)_5.0T_0.438K_90deg_Tdep_raw_.dat", "IDS0343_210904_RAW_cal_CeCoIn5_4th_072_C(f)_5.0T_0.53K_90deg_Tdep_raw_.dat", "IDS0344_210904_RAW_cal_CeCoIn5_4th_073_C(f)_5.0T_0.62K_90deg_Tdep_raw_.dat"]
  in  "tab 5":enum32{"Page 1"}(tab)
  in  "Math→τ! :q":bool
  in  "ω0 (rad/sec)":dbl(slide)=19.063235402868393 scale=0.001..50000.0 scale format="%#_2p"
  in  "offset Re\noffset Im":cluster{"Numeric":dbl, "Numeric":dbl}(slide)={"Numeric"=-62465346.53465346, "Numeric"=0.0} scale=-70000000.0..500000.0 scale format="%#_1p"
  in  "tab 44":enum32{"default values "}(tab)
  in  "default selector":T14(array[cluster])=[{"Plost: sweep window"=enum."ζ", "used default"=FALSE}, {"Plost: sweep window"=enum."τ1", "used default"=FALSE}, {"Plost: sweep window"=enum."τS", "used default"=FALSE}, {"Plost: sweep window"=enum."τN", "used default"=FALSE}, {"Plost: sweep window"=enum."τC", "used default"=FALSE}, {"Plost: sweep window"=enum."κ0", "used default"=FALSE}]
  in  "default values string":string="\"0\"->   <|\"T\" -> 0.120000, \"τN\"-> 0.670097, \"τC\"-> 0.001215, \"ζ\"-> 0.368640, \"κ0\"-> 0.00000000044100|>   ,\n\"1\"->   <|\"T\" -> 0.220000, \"τN\"-> 0.057428, \"τC\"-> 0.001386, \"ζ\"-> 0.131633, \"κ0\"-> 0.00000000120283|>   ,\n\"2\"->   <|\"T\" -> 0.320000, \"τN\"-> 0.014576, \"τC\"-> 0.001971, \"ζ\"-> 0.063259, \"κ0\"-> 0.00000000186767|>   ,\n\"3\"->   <|\"T\" -> 0.420000, \"τN\"-> 0.005816, \"τC\"-> 0.002645, \"ζ\"-> 0.041943, \"κ0\"-> 0.00000000259214|>   ,\n\"4\"->   <|\"T\" -> 0.520000, \"τN\"-> 0.002807, \"τC\"-> 0.003188, \"ζ\"-> 0.030182, \"κ0\"-> 0.00000000339327|>   ,\n\"5\"->   <|\"T\" -> 0.620000, \"τN\"-> 0.001928, \"τC\"-> 0.003634, \"ζ\"-> 0.025126, \"κ0\"-> 0.00000000404950|>   ,\n\"6\"->   <|\"T\" -> 0.720000, \"τN\"-> 0.001251, \"τC\"-> 0.004021, \"ζ\"-> 0.023386, \"κ0\"-> 0.00000000484450|>   ,\n\"7\"->   <|\"T\" -> 0.820000, \"τN\"-> 0.000866, \"τC\"-> 0.004389, \"ζ\"-> 0.022054, \"κ0\"-> 0.00000000563624|>   ,\n\"8\"->   <|\"T\" -> 0.920000, \"τN\"-> 0.000673, \"τC\"-> 0.004723, \"ζ\"-> 0.021623, \"κ0\"-> 0.00000000639866|>   ,\n\"9\"->   <|\"T\" -> 1.020000, \"τN\"-> 0.000537, \"τC\"-> 0.005044, \"ζ\"-> 0.021243, \"κ0\"-> 0.00000000716107|>   ,\n\"10\"->   <|\"T\" -> 1.120000, \"τN\"-> 0.000431, \"τC\"-> 0.005344, \"ζ\"-> 0.020967, \"κ0\"-> 0.00000000793323|>   ,\n\"11\"->   <|\"T\" -> 1.220000, \"τN\"-> 0.000336, \"τC\"-> 0.005596, \"ζ\"-> 0.020955, \"κ0\"-> 0.00000000874437|>   ,\n\"12\"->   <|\"T\" -> 1.320000, \"τN\"-> 0.000267, \"τC\"-> 0.005838, \"ζ\"-> 0.020944, \"κ0\"-> 0.00000000955551|>   ,\n\"13\"->   <|\"T\" -> 1.420000, \"τN\"-> 0.000216, \"τC\"-> 0.006071, \"ζ\"-> 0.020934, \"κ0\"-> 0.00000001036666|>   ,\n\"14\"->   <|\"T\" -> 1.520000, \"τN\"-> 0.000177, \"τC\"-> 0.006297, \"ζ\"-> 0.020925, \"κ0\"-> 0.00000001117780|>   ,\n\"15\"->   <|\"T\" -> 1.620000, \"τN\"-> 0.000147, \"τC\"-> 0.006517, \"ζ\"-> 0.020916, \"κ0\"-> 0.00000001198894|>   ,\n\"16\"->   <|\"T\" -> 1.720000, \"τN\"-> 0.000123, \"τC\"-> 0.006730, \"ζ\"-> 0.020907, \"κ0\"-> 0.00000001280009|>   ,\n\"17\"->   <|\"T\" -> 1.820000, \"τN\"-> 0.000105, \"τC\"-> 0.006885, \"ζ\"-> 0.020876, \"κ0\"-> 0.00000001362415|>   ,\n\"18\"->   <|\"T\" -> 1.920000, \"τN\"-> 0.000091, \"τC\"-> 0.006831, \"ζ\"-> 0.020754, \"κ0\"-> 0.00000001449990|>   ,\n\"19\"->   <|\"T\" -> 2.020000, \"τN\"-> 0.000080, \"τC\"-> 0.006781, \"ζ\"-> 0.020639, \"κ0\"-> 0.00000001537565|>   ,\n\"20\"->   <|\"T\" -> 2.120000, \"τN\"-> 0.000070, \"τC\"-> 0.006733, \"ζ\"-> 0.020530, \"κ0\"-> 0.00000001625140|>   ,\n\"21\"->   <|\"T\" -> 2.220000, \"τN\"-> 0.000062, \"τC\"-> 0.006687, \"ζ\"-> 0.020427, \"κ0\"-> 0.00000001712715|>   ,\n\"22\"->   <|\"T\" -> 2.320000, \"τN\"-> 0.000056, \"τC\"-> 0.006644, \"ζ\"-> 0.020329, \"κ0\"-> 0.00000001800290|>   ,\n\"23\"->   <|\"T\" -> 2.420000, \"τN\"-> 0.000050, \"τC\"-> 0.006603, \"ζ\"-> 0.020235, \"κ0\"-> 0.00000001887865|>   ,\n\"24\"->   <|\"T\" -> 2.520000, \"τN\"-> 0.000045, \"τC\"-> 0.006564, \"ζ\"-> 0.020146, \"κ0\"-> 0.00000001975440|>   ,\n\"25\"->   <|\"T\" -> 2.620000, \"τN\"-> 0.000040, \"τC\"-> 0.006527, \"ζ\"-> 0.020060, \"κ0\"-> 0.00000002063015|>   ,\n\"26\"->   <|\"T\" -> 2.720000, \"τN\"-> 0.000037, \"τC\"-> 0.006491, \"ζ\"-> 0.019978, \"κ0\"-> 0.00000002150590|>   ,\n\"27\"->   <|\"T\" -> 2.820000, \"τN\"-> 0.000033, \"τC\"-> 0.006457, \"ζ\"-> 0.019899, \"κ0\"-> 0.00000002238165|>   ,\n\"28\"->   <|\"T\" -> 2.920000, \"τN\"-> 0.000030, \"τC\"-> 0.006424, \"ζ\"-> 0.019824, \"κ0\"-> 0.00000002325740|>   ,\n\"29\"->   <|\"T\" -> 3.020000, \"τN\"-> 0.000028, \"τC\"-> 0.006374, \"ζ\"-> 0.019852, \"κ0\"-> 0.00000002421662|>   ,\n\"30\"->   <|\"T\" -> 3.120000, \"τN\"-> 0.000026, \"τC\"-> 0.006255, \"ζ\"-> 0.020282, \"κ0\"-> 0.00000002550973|>   ,\n\"31\"->   <|\"T\" -> 3.220000, \"τN\"-> 0.000024, \"τC\"-> 0.006143, \"ζ\"-> 0.020708, \"κ0\"-> 0.00000002680284|>   ,\n\"32\"->   <|\"T\" -> 3.320000, \"τN\"-> 0.000023, \"τC\"-> 0.006036, \"ζ\"-> 0.021130, \"κ0\"-> 0.00000002809596|>   ,\n\"33\"->   <|\"T\" -> 3.420000, \"τN\"-> 0.000021, \"τC\"-> 0.005933, \"ζ\"-> 0.021547, \"κ0\"-> 0.00000002938907|>   ,\n\"34\"->   <|\"T\" -> 3.520000, \"τN\"-> 0.000020, \"τC\"-> 0.005836, \"ζ\"-> 0.021960, \"κ0\"-> 0.00000003068218|>   ,\n\"35\"->   <|\"T\" -> 3.620000, \"τN\"-> 0.000019, \"τC\"-> 0.005742, \"ζ\"-> 0.022368, \"κ0\"-> 0.00000003197529|>   ,\n\"36\"->   <|\"T\" -> 3.720000, \"τN\"-> 0.000018, \"τC\"-> 0.005653, \"ζ\"-> 0.022774, \"κ0\"-> 0.00000003326840|>   ,\n\"37\"->   <|\"T\" -> 3.820000, \"τN\"-> 0.000017, \"τC\"-> 0.005567, \"ζ\"-> 0.023175, \"κ0\"-> 0.00000003456151|>   ,\n\"38\"->   <|\"T\" -> 3.920000, \"τN\"-> 0.000016, \"τC\"-> 0.005485, \"ζ\"-> 0.023573, \"κ0\"-> 0.00000003585462|>   ,\n\"39\"->   <|\"T\" -> 4.020000, \"τN\"-> 0.000015, \"τC\"-> 0.005406, \"ζ\"-> 0.023967, \"κ0\"-> 0.00000003714773|>   ,\n\"40\"->   <|\"T\" -> 4.120000, \"τN\"-> 0.000014, \"τC\"-> 0.005330, \"ζ\"-> 0.024358, \"κ0\"-> 0.00000003844084|>   ,\n\"41\"->   <|\"T\" -> 4.220000, \"τN\"-> 0.000013, \"τC\"-> 0.005257, \"ζ\"-> 0.024746, \"κ0\"-> 0.00000003973396|>   ,\n\"42\"->   <|\"T\" -> 4.320000, \"τN\"-> 0.000013, \"τC\"-> 0.005186, \"ζ\"-> 0.025131, \"κ0\"-> 0.00000004102707|>   ,\n\"43\"->   <|\"T\" -> 4.420000, \"τN\"-> 0.000012, \"τC\"-> 0.005118, \"ζ\"-> 0.025512, \"κ0\"-> 0.00000004232018|>   ,\n\"44\"->   <|\"T\" -> 4.520000, \"τN\"-> 0.000012, \"τC\"-> 0.005053, \"ζ\"-> 0.025891, \"κ0\"-> 0.00000004361329|>   ,\n\"45\"->   <|\"T\" -> 4.620000, \"τN\"-> 0.000011, \"τC\"-> 0.004990, \"ζ\"-> 0.026267, \"κ0\"-> 0.00000004490640|>   ,\n\"46\"->   <|\"T\" -> 4.720000, \"τN\"-> 0.000011, \"τC\"-> 0.004928, \"ζ\"-> 0.026640, \"κ0\"-> 0.00000004619951|>   ,\n\"47\"->   <|\"T\" -> 4.820000, \"τN\"-> 0.000010, \"τC\"-> 0.004869, \"ζ\"-> 0.027010, \"κ0\"-> 0.00000004749262|>   ,\n\"48\"->   <|\"T\" -> 4.920000, \"τN\"-> 0.000010, \"τC\"-> 0.004812, \"ζ\"-> 0.027378, \"κ0\"-> 0.00000004878573|>   ,"
  in  "load default values":bool
  in  "selector":T15={"ignore set of !"=FALSE, "set (1T|2B)"=0, "ignore side !"=FALSE, "side (8S|4R)"=0, "ignore θ !"=FALSE, "ignore B !"=FALSE, "T (K)"=10, "ignore T !"=TRUE, "θ (deg)"=4, "B (T)"=3, "lookup"={"set of lookup"={0=1.0, 1=2.0}, "all set of"={1.0, 2.0}, "T lookup"={0=0.12, 1=0.122, 2=0.14, 3=0.148, 4=0.15, 5=0.157, 6=0.16, 7=0.168, 8=0.17, 9=0.178, 10=0.179, 11=0.197, 12=0.2, 13=0.22, 14=0.249, 15=0.25, 16=0.255, 17=0.26, 18=0.28, 19=0.3, 20=0.307, 21=0.308, 22=0.31, 23=0.33, 24=0.36, 25=0.4, 26=0.43, 27=0.438, 28=0.48, 29=0.512, 30=0.53, 31=0.58, 32=0.61, 33=0.62, 34=0.63, 35=0.677, 36=0.68, 37=0.81, 38=0.83, 39=0.91, 40=1.0, 41=1.1, 42=1.13, 43=1.23, 44=1.25, 45=1.31, 46=1.39, 47=1.52, 48=1.55, 49=1.8, 50=1.9, 51=1.97, 52=3.0, 53=3.1, 54=3.11, 55=3.19, 56=5.7, 57=5.75, 58=5.8}, "θ lookup"={0=0.0, 1=30.0, 2=45.0, 3=60.0, 4=90.0}, "B lookup"={0=0.0, 1=1.0, 2=2.0, 3=5.0, 4=6.0, 5=7.0, 6=8.0, 7=9.0, 8=10.0, 9=11.0, 10=12.0}, "all T's"={0.12, 0.122, 0.14, 0.148, 0.15, 0.157, 0.16, 0.168, 0.17, 0.178, 0.179, 0.197, 0.2, 0.22, 0.249, 0.25, 0.255, 0.26, 0.28, 0.3, 0.307, 0.308, 0.31, 0.33, 0.36, 0.4, 0.43, 0.438, 0.48, 0.512, 0.53, 0.58, 0.61, 0.62, 0.63, 0.677, 0.68, 0.81, 0.83, 0.91, 1.0, 1.1, 1.13, 1.23, 1.25, 1.31, 1.39, 1.52, 1.55, 1.8, 1.9, 1.97, 3.0, 3.1, 3.11, 3.19, 5.7, 5.75, 5.8}, "all θ's"={0.0, 30.0, 45.0, 60.0, 90.0}, "all B's"={0.0, 1.0, 2.0, 5.0, 6.0, 7.0, 8.0, 9.0, 10.0, 11.0, 12.0}, "all sides"={4000.0, 8000.0}, "side lookup"={0=4000.0, 1=8000.0}}} {"B (T)" items=["0.000", "1.000", "2.000", "5.000", "6.000", "7.000", "8.000", "9.000", "10.000", "11.000", "12.000"]; "θ (deg)" items=["0.000", "30.000", "45.000", "60.000", "90.000"]; "T (K)" items=["0.120", "0.122", "0.140", "0.148", "0.150", "0.157", "0.160", "0.168", "0.170", "0.178", "0.179", "0.197", "0.200", "0.220", "0.249", "0.250", "0.255", "0.260", "0.280", "0.300", "0.307", "0.308", "0.310", "0.330", "0.360", "0.400", "0.430", "0.438", "0.480", "0.512", "0.530", "0.580", "0.610", "0.620", "0.630", "0.677", "0.680", "0.810", "0.830", "0.910", "1.000", "1.100", "1.130", "1.230", "1.250", "1.310", "1.390", "1.520", "1.550", "1.800", "1.900", "1.970", "3.000", "3.100", "3.110", "3.190", "5.700", "5.750", "5.800"]; "side (8S|4R)" items=["4000", "8000"]; "set (1T|2B)" items=["1", "2"]}
  in  "parameter selectors tab":enum32{"Page 1"}(tab)
  in  "colors":u32[](array[colorbox])=[7087058, 56538, 2062078, 16740827, 16755712, 11121611, 8285330, 9272482, 9204890]
  in  "parameter":T4[](array[typedef])=[enum."ζ", enum."τ1", enum."τS", enum."τN", enum."τC", enum."κ0"]
  in  "overwrite offset":bool=TRUE
  in  "landscape plots":enum32{"Page 1", "Page 2"}(tab)
  in  "range one":dbl(slide)=0.006965 min=0.0 max=0.3 step=1e-06 scale=0.0001..1.0 scale format="%#_3p"
  in  "one":T4=enum."τS"
  out "Plot: goodness":cluster{"Freq out (Hz)":dbl[], dbl[]}[](graph)
  in  "plot landscape!":bool
  in  "range two":dbl(slide)=0.0039049999999999996 min=0.0 max=0.3 step=1e-06 scale=0.0001..1.0 scale format="%#_3p"
  in  "two":T4=enum."τ1"
  in  "what":enum16{"1d plots", "2d plots "}(ring)
  in  "# points":i32=200
  in  "Array":T4[](array[typedef])=[enum."ζ", enum."τ1", enum."τS", enum."τN", enum."τC"]
  in  "color Map":map{T4, u32}(c390)={enum."ζ"=7087058, enum."τ1"=56538, enum."τS"=2062078, enum."τN"=16740827, enum."τC"=16755712, enum."κ0"=11121611}
